vi "number4-insertion sorting.vi"() -> ()   [LabVIEW 2014]
panel:
  out "Waveform Graph":dbl[](graph)
  out "After insertion sort":dbl[](array[numeric])
  out "before insertion sort":dbl[](array[numeric])
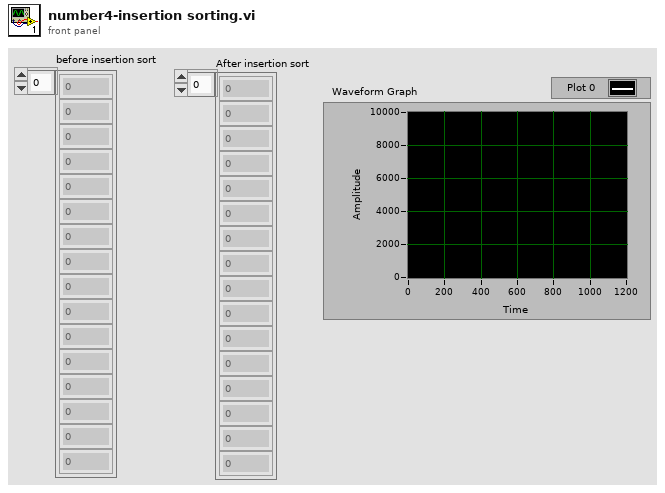
[diagram p1: front panel]
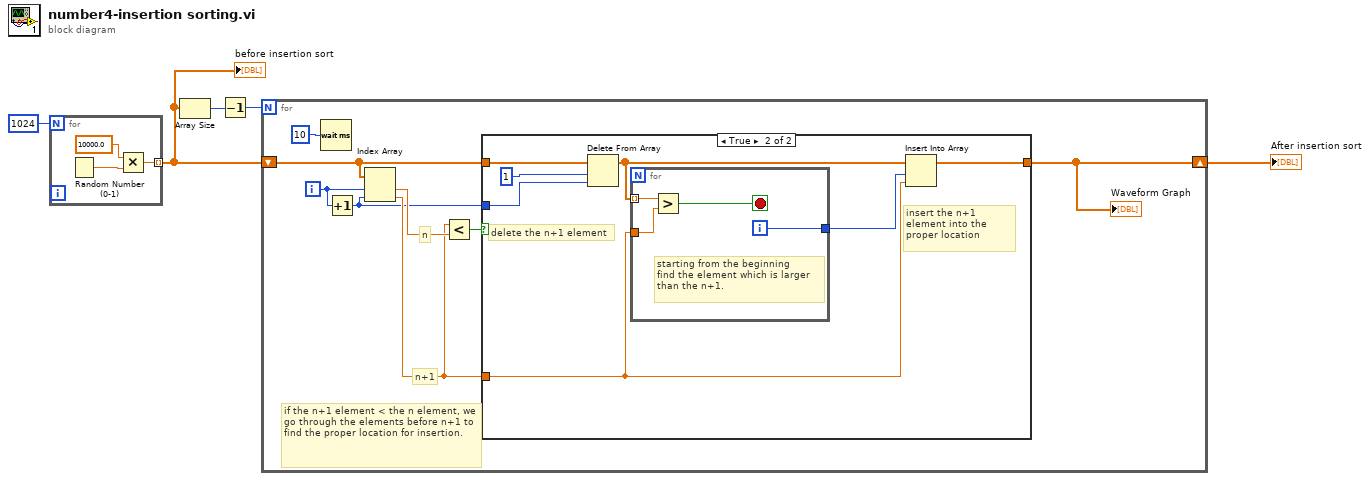
[diagram p0: block diagram]
diagram:
  n1 = for {
    N: 1024 -> [_]
    tunnel: [w6] -> w4 mode=indexing
    n2 = Random Number (0-1)() -> (number: 0 to 1=w8:dbl)
    n3 = Multiply(x=10000.0, y=w8) -> (x*y=w6:dbl)
  }
  "before insertion sort" <- w4
  n4 = Array Size(array=w4) -> (size(s)=w3:i32)
  n5 = Decrement(x=w3) -> (x-1=w2:i32)
  n6 = for {
    N: w2 -> [_]
    shift-right: [w10] -> w1
    shift-left: w4 -> [w15]
    i -> [w12]
    # "if the n+1 element < the n element, we go through the elements before n+1 to find the proper location for insertion."
    # "n+1"
    # "n"
    n7 = Wait (ms)(milliseconds to wait=u32 10) -> ()  [unwired: 1 out]
    n8 = Increment(x=w12) -> (x+1=w11:i32)
    n9 = Index Array(array=w15, index #1=w12, index #2=w11) -> (element #1=w14:dbl, element #2=w13:dbl)
    n10 = Less?(x=w13, y=w14) -> (x < y?=w16:bool)
    n11 = case shown="True" w16 {
      tunnel: w15 -> [w17 w24]
      tunnel: [w17 w20] -> w10
      tunnel: w11 -> [_ w22]
      tunnel: w13 -> [_ w21]
      frame False {
      }
      frame True {
        # "insert the n+1 element into the proper location"
        # "delete the n+1 element"
        n12 = Delete From Array(array=w24, length=1 ("index"), index=w22) -> (array with subset deleted=w19:dbl[])  [unwired: 1 out]
        n13 = for {
          tunnel: w21 -> [w28]
          tunnel: [w26] -> w18
          tunnel: w19 -> [w25] mode=indexing
          i -> [w26]
          stop <- w27 stop-if-true
          # "starting from the beginning\nfind the element which is larger\nthan the n+1."
          n14 = Greater?(x=w25, y=w28) -> (0:w27:bool)
        }
        n15 = Insert Into Array(array=w19, index=w18, new element=w21) -> (w20:dbl[])
      }
    }
    "Waveform Graph" <- w10
  }
  "After insertion sort" <- w1
